vi "SingleToU8ArrayBigEndian(SubVI).vi"(11 "long data":sgl) -> (1 "third byte":u8, 2 "send byte":u8, 3 "first byte":u8, 4 "forth byte":u8)   [LabVIEW 2012]
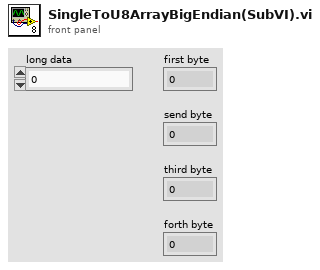
[diagram p1: front panel]
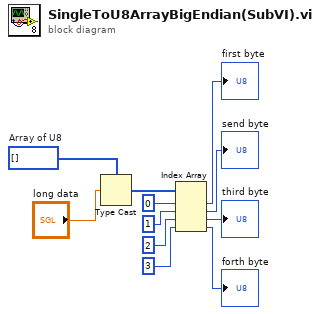
[diagram p0: block diagram]
diagram:
  w5 = u8[] []  # Array of U8
  n1 = Type Cast(type=w5, x="long data") -> (*(type *) &x=w6:u8[])
  n2 = Index Array(array=w6, index #1=0, index #2=1, index #3=2, index #4=3) -> (element #1=→"first byte":u8, element #2=→"send byte":u8, element #3=→"third byte":u8, element #4=→"forth byte":u8)
